vi "UTC Timestamp.vi"() -> ()   [LabVIEW 2016]
panel:
  out "Time Stamp":timestamp
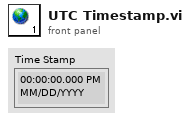
[diagram p1: front panel]
diagram:
